vi "Autoadjust.vi"(7 "Adjustment Rate":dbl=0.01, 8 "error in (no error)":errorcluster, 10 "Fixated":bool, 11 "TrialBasedExperiment in":refnum<class "TrialBasedExperiment.lvclass">) -> (0 "error out":errorcluster, 3 "TrialBasedExperiment out":refnum<class "TrialBasedExperiment.lvclass">)   [LabVIEW 2014, in "AcquisitionCoreObjects.lvlib" / "TrialBasedExperiment.lvclass"]
uses:
  TrialBasedExperiment.lvclass
  <vilib>/Analysis/NI_AALBase.lvlib
panel:
  out "size(s)":i32
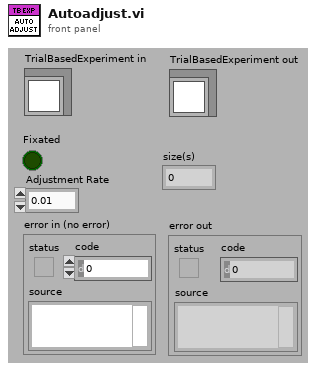
[diagram p1: front panel]
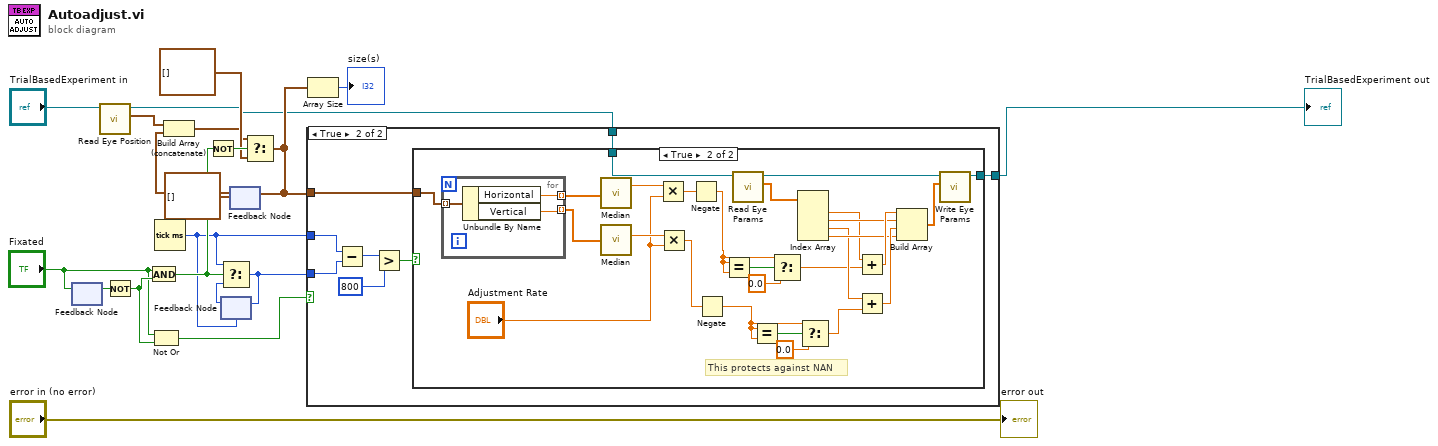
[diagram p0: block diagram]
diagram:
  n1 = feedback-in #1("Fixated") -> ()
  n2 = feedback #1() -> (w18:bool)  [unwired: 1 in]
  n3 = call-dynamic "Read Eye Position.vi"("TrialBasedExperiment in"="TrialBasedExperiment in") -> ("Eye Position"=w10:cluster{"Horizontal":dbl, "Vertical":dbl}, "TrialBasedExperiment out"=w2:refnum<class "TrialBasedExperiment.lvclass">)  [unwired: 8 in, 1 out]
  n4 = Not(x=w18) -> (.not. x?=w17:bool)
  n5 = And(x="Fixated", y=w17) -> (x .and. y?=w11:bool)
  n6 = Not Or(1:w17, 2:"Fixated") -> (0:w15:bool)
  n7 = Tick Count (ms)() -> (millisecond timer value=w3:u32)
  n8 = Not(x=w11) -> (.not. x?=w12:bool)
  n9 = feedback #2(w3) -> (w19:u32)
  n10 = Select(t=w3, s=w11, f=w19) -> (s? t:f=w14:u32)
  n11 = feedback-in #2(w14) -> ()
  n12 = feedback #3(cluster{"Horizontal":dbl, "Vertical":dbl}[] [] ("t")) -> (w9:cluster{"Horizontal":dbl, "Vertical":dbl}[])
  n13 = Build Array (concatenate)(w10, w9) -> (w7:cluster{"Horizontal":dbl, "Vertical":dbl}[])
  n14 = Select(t=w7, s=w12, f=cluster{"Horizontal":dbl, "Vertical":dbl}[] [] ("t")) -> (s? t:f=w6:cluster{"Horizontal":dbl, "Vertical":dbl}[])
  n15 = feedback-in #3(w6) -> ()
  n16 = case shown="True" w15 {
    tunnel: w3 -> [_ w29]
    tunnel: w14 -> [_ w28]
    tunnel: w6 -> [_ w24]
    tunnel: w2 -> [w21 w23]
    tunnel: [w21 w22] -> w1
    frame False {
    }
    frame True {
      n17 = Subtract(x=w29, y=w28) -> (x-y=w27:u32)
      n18 = Greater?(x=w27, y=u32 800) -> (0:w25:bool)
      n19 = case shown="True" w25 {
        tunnel: w24 -> [_ w57]
        tunnel: w23 -> [w30 w43]
        tunnel: [w30 w41] -> w22
        frame False {
        }
        frame True {
          # "This protects against NAN"
          n20 = for {
            tunnel: w57 -> [w60] mode=indexing
            tunnel: [w59] -> w56 mode=indexing
            tunnel: [w58] -> w55 mode=indexing
            n21 = Unbundle By Name(w60) -> ("Horizontal"=w59:dbl, "Vertical"=w58:dbl)
          }
          n22 = call <vilib>:"Median.vi"("X"=w56) -> ("median"=w53:dbl)  [unwired: 1 out]
          n23 = call <vilib>:"Median.vi"("X"=w55) -> ("median"=w54:dbl)  [unwired: 1 out]
          n24 = Multiply(x=w53, y="Adjustment Rate") -> (x*y=w34:dbl)
          n25 = Multiply(x=w54, y="Adjustment Rate") -> (x*y=w32:dbl)
          n26 = Negate(x=w34) -> (-x=w33:dbl)
          n27 = Negate(x=w32) -> (-x=w31:dbl)
          n28 = Equal?(x=w33, y=w33) -> (x = y?=w40:bool)
          n29 = call-dynamic "Read Eye Params.vi"("TrialBasedExperiment in"=w43) -> ("Eye Params"=w44:dbl[], "TrialBasedExperiment out"=w42:refnum<class "TrialBasedExperiment.lvclass">)  [unwired: 8 in, 1 out]
          n30 = Equal?(x=w31, y=w31) -> (x = y?=w37:bool)
          n31 = Select(t=w33, s=w40, f=0.0) -> (s? t:f=w38:dbl)
          n32 = Index Array(array=w44) -> (element #1=w45:dbl, element #2=w48:dbl, element #3=w46:dbl, element #4=w47:dbl)  [unwired: 4 in]
          n33 = Select(t=w31, s=w37, f=0.0) -> (s? t:f=w35:dbl)
          n34 = Add(x=w45, y=w38) -> (x+y=w50:dbl)
          n35 = Add(x=w46, y=w35) -> (x+y=w49:dbl)
          n36 = Build Array(w50, w48, w49, w47) -> (w51:dbl[])
          n37 = call-dynamic "Write Eye Params.vi"("Eye Params"=w51, "TrialBasedExperiment in"=w42) -> ("TrialBasedExperiment out"=w41:refnum<class "TrialBasedExperiment.lvclass">)  [unwired: 8 in, 1 out]
        }
      }
    }
  }
  "TrialBasedExperiment out" <- w1
  n38 = Array Size(array=w6) -> (size(s)=→"size(s)":i32)
  "error out" <- "error in (no error)"
